vi "Set or Reset Digital IO Pins.vi"(8 "error in (no error)":errorcluster, 9 "Digital IO Line (T: Bit High)":bool=TRUE, 10 "Digital IO Line (1)":u32=1, 11 "VISA resource name":refnum<visa-resource-name>) -> (0 "error out":errorcluster, 3 "VISA resource name out":refnum<visa-resource-name>)   [LabVIEW 2020, in "Keithley 2450.lvlib"]
doc: "Sets a digital I/O line high or low."
uses:
  <instrlib>/Keithley 2450/Keithley 2450.lvlib
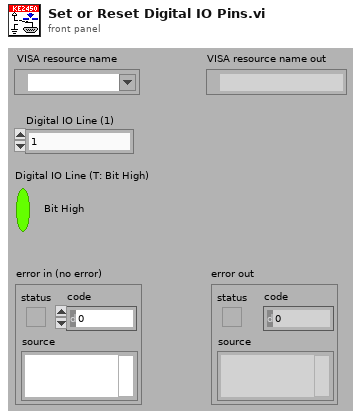
[diagram p1: front panel]
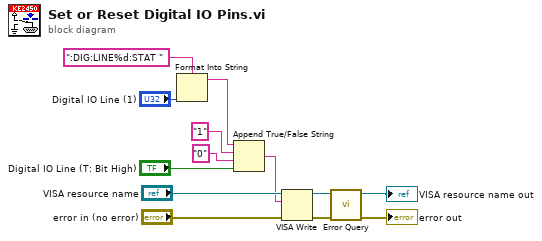
[diagram p0: block diagram]
diagram:
  n1 = Format Into String(format string=":DIG:LINE%d:STAT ", "Digital IO Line (1)") -> (resulting string=w5:string)  [unwired: 2 in, 1 out]
  n2 = Append True/False String(1:"Digital IO Line (T: Bit High)", 2:"0" ("false string"), 3:"1" ("true string"), 4:w5) -> (0:w1:string)
  n3 = VISA Write(VISA resource name="VISA resource name", write buffer=w1, error in (no error)="error in (no error)") -> (VISA resource name out=w11:refnum<visa-resource-name>, error out=w8:errorcluster)  [unwired: 1 out]
  n4 = call <instrlib>:"Error Query.vi"("error in (no error)"=w8, "VISA resource name"=w11) -> ("error out"=→"error out":errorcluster, "VISA resource name out"=→"VISA resource name out":refnum<visa-resource-name>)  [unwired: 8 out]
